vi "Get Name.vi"(8 "error in (no error)":errorcluster, 11 "Button in":refnum<class "Button.lvclass">) -> (0 "error out":errorcluster, 2 "Name":string, 3 "Button out":refnum<class "Button.lvclass">)   [LabVIEW 2020, in "Button.lvlib" / "Button.lvclass"]
uses:
  Button.lvclass
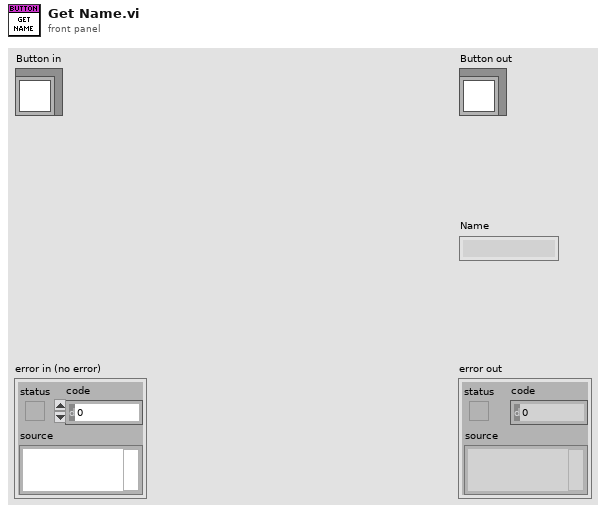
[diagram p1: front panel]
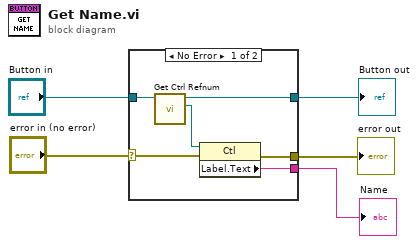
[diagram p0: block diagram]
diagram:
  n1 = case shown="No Error" "error in (no error)" {
    selector: "error in (no error)" -> [w7 w13]
    tunnel: "Button in" -> [w11 w12]
    tunnel: [w6 w13] -> w3
    tunnel: [w10 w12] -> w2
    tunnel: [w8 _] -> w1
    frame No Error {
      n2 = call-dynamic "Get Ctrl Refnum.vi"("Button in"=w11) -> ("Ctl Refnum"=w9:refnum<vi>, "Button out"=w10:refnum<class "Button.lvclass">)  [unwired: 8 in, 1 out]
      n3 = property class="Ctl"(reference=w9, error in=w7) -> (error out=w6:errorcluster, "Label.Text"=w8:string)  [unwired: 1 out]
    }
    frame Error {
    }
  }
  "error out" <- w3
  "Button out" <- w2
  "Name" <- w1
